vi "ContMainInit.vi"(8 "ion coords":T1={"Top :"=103.0, "Bottom :"=100.0, "Left :"=100.0, "Right :"=103.0}, 9 "configuration file path":path, 10 "File Paths":T2={"Local Save Path"=path "\\\\smbhome.uscs.susx.ac.uk\\cv222/Desktop/data", "Newton Save Path"=path "Z:/#Projects/Entanglement/data", "File Name"="test", "LocalSave"=TRUE}, 11 "Compiler Settings":T3={"Python Path"=path "", "Main File"="", "Meta File"="", "Aux File"="", "Pre File"="metascript.txt"}) -> (2 "kinetic img size":cluster{"xpixels":i32, "ypixels":i32}, 3 "steps":dbl)   [LabVIEW 2019]
uses:
  PulseCompiler/CompilerSettings.ctl
  controls/FilePaths.ctl
  Camera/CameraCoordsControl.ctl
  controls/GlobalExp.vi
  Global.lvlib
panel:
  in  "ion coords 2":T1={"Top :"=103.0, "Bottom :"=100.0, "Left :"=100.0, "Right :"=103.0}
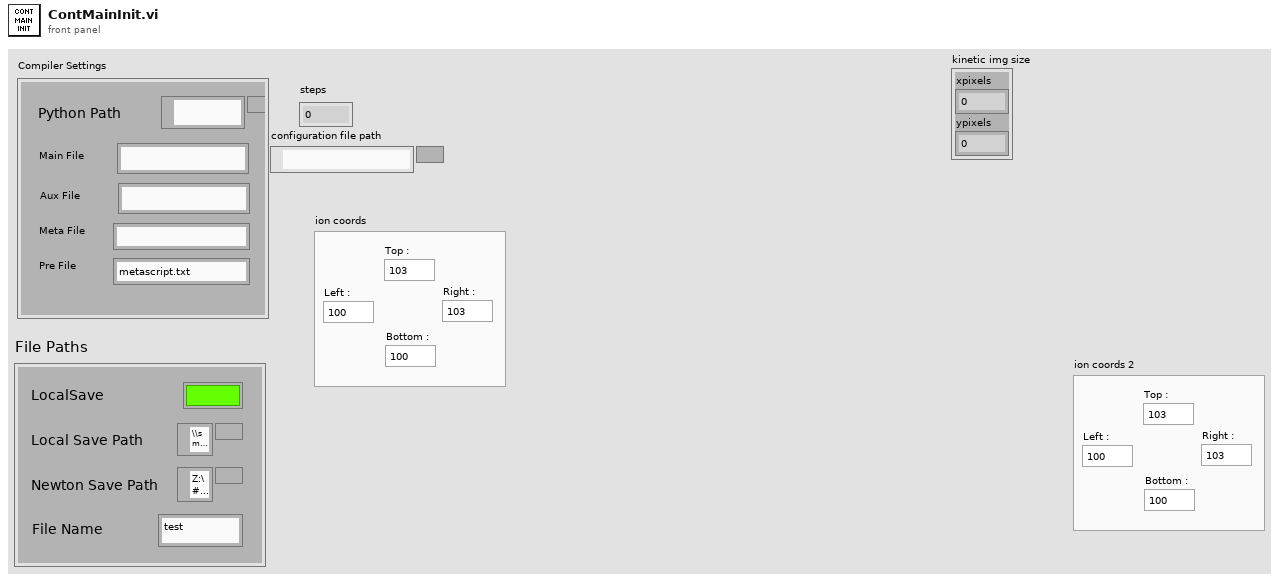
[diagram p1: front panel]
types:
  T1 = typedef "CameraCoordsControl.ctl" = cluster{"Top :":dbl, "Bottom :":dbl, "Left :":dbl, "Right :":dbl}
  T2 = typedef "FilePaths.ctl" = cluster{"Local Save Path":path, "Newton Save Path":path, "File Name":string, "LocalSave":bool}
  T3 = typedef "CompilerSettings.ctl" = cluster{"Python Path":path, "Main File":string, "Meta File":string, "Aux File":string, "Pre File":string}
  T4 = typedef "Params.ctl" = cluster{"steps":i16, "runs":i16, "comment":string, "mathematica":string, "calib":i8, "logmsg":string, "ndets":i16}
  T5 = cluster{"Sequence Exposure Time (secs)":sgl, "# of kinetics":i32, "triggered?":bool}
  T6 = typedef "MasterExpControl.ctl" = cluster{"Main Steps":dbl, "Main Runs":dbl, "ExpStatus":enum16{"Innit", "Stop", "Idle", "MainRunning", "AuxRunning"}, "Main Current Step":dbl, "ExpNum":dbl, "NewData":bool, "date":string, "command":string, "Stop":bool, "Pause":bool, "Mathematica":string, "Main/Meta":bool, "UpdateMath":bool, "Camera":bool, "MetaExpOver":bool, "NextMetaExp":bool}
  T7 = cluster{"x":i32, "width":i32, "y":i32, "height":i32}
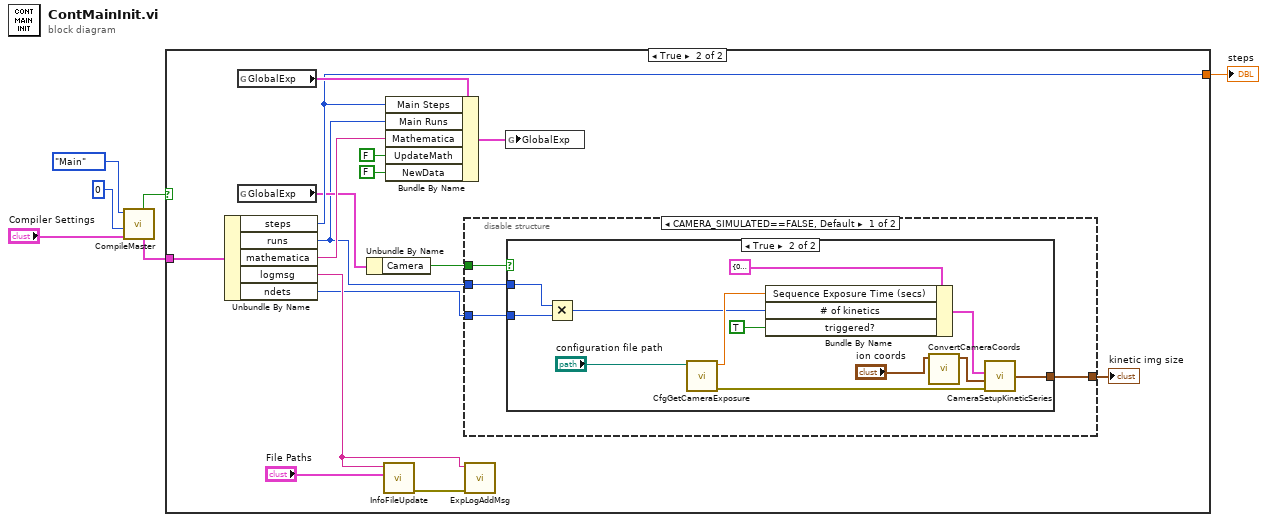
[diagram p0: block diagram]
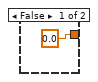
[diagram p2: hidden frame]
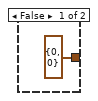
[diagram p3: hidden frame]
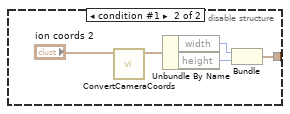
[diagram p4: hidden frame]
diagram:
  n1 = call "CompileMaster.vi"("Type"=enum16{"Meta", "Aux", "Main"}."Main", "Stepnum"=0, "Compiler Settings"="Compiler Settings") -> ("CompileSuccess?"=w5:bool, "Params"=w4:T4)  [unwired: 1 in, 4 out]
  n2 = case shown="True" w5 {
    tunnel: w4 -> [_ w22]
    tunnel: [0.0 ("steps") w17] -> w6
    frame False {
    }
    frame True {
      n3 = Unbundle By Name(w22) -> ("steps"=w17:i16, "runs"=w12:i16, "mathematica"=w18:string, "logmsg"=w15:string, "ndets"=w11:i16)
      n4 = global read "GlobalExp.vi" "GlobalExp"() -> (w20:T6)
      n5 = global read "GlobalExp.vi" "GlobalExp"() -> (w14:T6)
      n6 = Unbundle By Name(w14) -> ("Camera"=w13:bool)
      n7 = call "InfoFileUpdate.vi"("File Paths"="File Paths", "info msg"=w15) -> ("error out"=w16:errorcluster)  [unwired: 9 in]
      n8 = Bundle By Name(cluster=w20, "Main Steps"=w17, "Main Runs"=w12, "Mathematica"=w18, "UpdateMath"=FALSE, "NewData"=FALSE) -> (w19:T6)
      n9 = disable-structure shown="CAMERA_SIMULATED==FALSE, Default" {
        disable-tunnel: w13 -> [w26 _]
        disable-tunnel: w12 -> [w25 _]
        disable-tunnel: w11 -> [w24 _]
        disable-tunnel: [w23 w40] -> w10
        frame condition #0 (active) {
          n10 = case shown="True" w26 {
            tunnel: w25 -> [_ w32]
            tunnel: w24 -> [_ w31]
            tunnel: [cluster{"xpixels":i32, "ypixels":i32} {"xpixels"=0, "ypixels"=0} ("image size") w29] -> w23
            frame False {
            }
            frame True {
              n11 = Multiply(x=w32, y=w31) -> (x*y=w30:i16)
              n12 = call "CfgGetCameraExposure.vi"("configuration file path"="configuration file path") -> ("error out"=w33:errorcluster, "cam exposure"=w36:dbl)  [unwired: 9 in]
              n13 = Bundle By Name(cluster=T5 {"Sequence Exposure Time (secs)"=0.0, "# of kinetics"=0, "triggered?"=FALSE} ("kinetic series pars"), "Sequence Exposure Time (secs)"=w36, "# of kinetics"=w30, "triggered?"=TRUE) -> (w38:T5)
              n14 = call "ConvertCameraCoords.vi"("ion coords"="ion coords") -> ("subimage cluster"=w34:T7)  [unwired: 10 in]
              n15 = call "CameraSetupKineticSeries.vi"("kinetic series pars"=w38, "subimage cluster"=w34, "error in (no error)"=w33) -> ("image size"=w29:cluster{"xpixels":i32, "ypixels":i32})  [unwired: 2 in, 2 out]
            }
          }
        }
        frame condition #1 {
          n16 = call "ConvertCameraCoords.vi"("ion coords"="ion coords 2") -> ("subimage cluster"=w43:T7)  [unwired: 10 in]
          n17 = Unbundle By Name(w43) -> ("width"=w42:i32, "height"=w41:i32)
          n18 = Bundle("width"=w42, "height"=w41) -> (w40:cluster{"width":i32, "height":i32})  [unwired: 1 in]
        }
      }
      "kinetic img size" <- w10
      n19 = call "ExpLogAddMsg.vi"("error in (no error)"=w16, "msg in"=w15) -> ()  [unwired: 9 in, 1 out]
      n20 = global write "GlobalExp.vi" "GlobalExp"(w19) -> ()
    }
  }
  "steps" <- w6
